vi "geve-generate_config_file.vi"(8 "error in (no error)":errorcluster) -> (0 "error out":errorcluster, 1 "serial cfg":T1={"timeout (ms)"=0, "VISA resource name"="", "baud rate"=0, "max expected byte count"=128}, 2 "info":string)   [LabVIEW 2018]
doc: "check if config file exists.\nif not create it ( also check if config folder exists) and populate default data.\nif exists, get the config."
uses:
  geve-serial_config_cluster.ctl
  <vilib>/Utility/config.llb/Write Key (String).vi
  <vilib>/Utility/config.llb/Write Key (I32).vi
  <vilib>/Utility/config.llb/Read Key (String).vi
  <vilib>/Utility/config.llb/Read Key (I32).vi
  <vilib>/Utility/config.llb/NI_LVConfig.lvlib
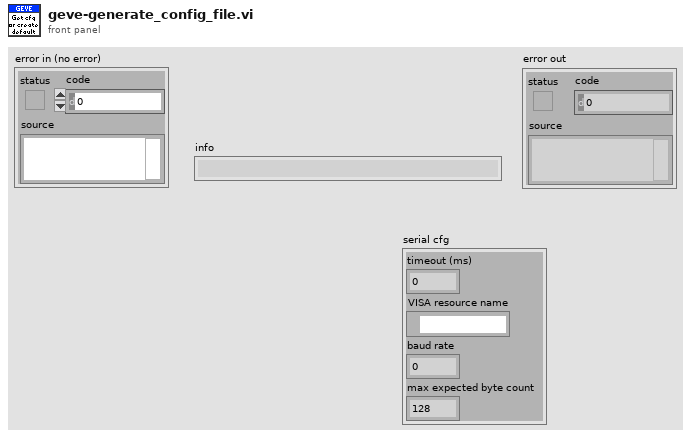
[diagram p1: front panel]
types:
  T1 = typedef "geve-serial_config_cluster.ctl" = cluster{"timeout (ms)":u32, "VISA resource name":refnum<visa-resource-name>, "baud rate":u32, "max expected byte count":u32}
  T2 = typedef "NI_LVConfig.lvlib/Config Data RefNum.ctl" = refnum<k1>
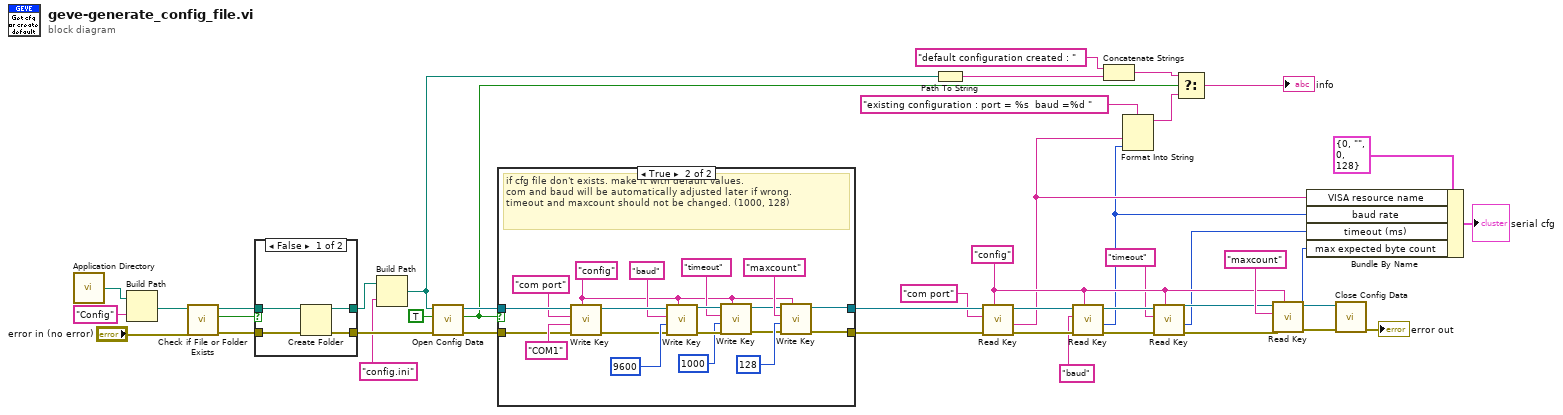
[diagram p0: block diagram]
diagram:
  w8 = "config" ("section")
  n1 = call <vilib>:"Application Directory.vi"() -> ("Application Directory"=w42:path)
  n2 = Build Path(base path=w42, name or relative path="Config") -> (appended path=w40:path)
  n3 = call <vilib>:"Check if File or Folder Exists.vi"("error in (no error)"="error in (no error)", "path"=w40) -> ("error out"=w35:errorcluster, "file or folder exists?"=w39:bool, "dup path"=w38:path)  [unwired: 7 in]
  n4 = case shown="False" w39 {
    tunnel: w38 -> [w47 w49]
    tunnel: [w46 w49] -> w26
    tunnel: [w44 w48] -> w36
    tunnel: w35 -> [w45 w48]
    frame False {
      n5 = Create Folder(path (use dialog)=w47, error in=w45) -> (created path=w46:path, error out=w44:errorcluster)  [unwired: 1 in, 1 out]
    }
    frame True {
    }
  }
  n6 = Build Path(base path=w26, name or relative path="config.ini") -> (appended path=w20:path)
  n7 = call <vilib>:"Open Config Data.vi"("error in (no error)"=w36, "create file if necessary (T)"=TRUE, "configuration file path"=w20) -> ("error out"=w33:errorcluster, "file created?"=w23:bool, "refnum"=w37:T2)  [unwired: 6 in]
  n8 = case shown="True" w23 {
    tunnel: w37 -> [w51 w70]
    tunnel: w33 -> [w50 w64]
    tunnel: [w51 w53] -> w31
    tunnel: [w50 w52] -> w30
    frame False {
    }
    frame True {
      w56 = "config" ("section")
      # "if cfg file don't exists. make it with default values.\ncom and baud will be automatically adjusted later if wrong.\ntimeout and maxcount should not be changed. (1000, 128)"
      n9 = call-poly <vilib>:"Write Key.vi"("section"=w56, "error in (no error)"=w64, "value"="COM1", "key"="com port", "refnum"=w70) -> ("error out"=w63:errorcluster, "refnum out"=w69:T2)  [unwired: 4 in, 1 out]
      n10 = call-poly <vilib>:"Write Key.vi"("section"=w56, "error in (no error)"=w63, "value"=9600, "key"="baud", "refnum"=w69) -> ("error out"=w61:errorcluster, "refnum out"=w62:T2)  [unwired: 4 in, 1 out]
      n11 = call-poly <vilib>:"Write Key.vi"("section"=w56, "error in (no error)"=w61, "value"=1000, "key"="timeout", "refnum"=w62) -> ("error out"=w55:errorcluster, "refnum out"=w54:T2)  [unwired: 4 in, 1 out]
      n12 = call-poly <vilib>:"Write Key.vi"("section"=w56, "error in (no error)"=w55, "value"=128, "key"="maxcount", "refnum"=w54) -> ("error out"=w52:errorcluster, "refnum out"=w53:T2)  [unwired: 4 in, 1 out]
    }
  }
  n13 = Path To String(path=w20) -> (string=w21:string)
  n14 = call-poly <vilib>:"Read Key.vi"("section"=w8, "error in (no error)"=w30, "key"="com port", "refnum"=w31) -> ("error out"=w29:errorcluster, "value"=w5:string, "refnum out"=w32:T2)  [unwired: 4 in, 1 out]
  n15 = call-poly <vilib>:"Read Key.vi"("section"=w8, "error in (no error)"=w29, "key"="baud", "refnum"=w32) -> ("error out"=w12:errorcluster, "value"=w4:i32, "refnum out"=w13:T2)  [unwired: 4 in, 1 out]
  n16 = Concatenate Strings("default configuration created : " ("section"), w21) -> (w19:string)
  n17 = Format Into String(format string="existing configuration : port = %s  baud =%d " ("section"), w5, w4) -> (resulting string=w17:string)  [unwired: 2 in, 1 out]
  n18 = call-poly <vilib>:"Read Key.vi"("section"=w8, "error in (no error)"=w12, "key"="timeout", "refnum"=w13) -> ("error out"=w11:errorcluster, "value"=w3:i32, "refnum out"=w14:T2)  [unwired: 4 in, 1 out]
  n19 = Select(t=w19, s=w23, f=w17) -> (s? t:f=→"info":string)
  n20 = call-poly <vilib>:"Read Key.vi"("section"=w8, "error in (no error)"=w11, "key"="maxcount", "refnum"=w14) -> ("error out"=w10:errorcluster, "value"=w2:i32, "refnum out"=w9:T2)  [unwired: 4 in, 1 out]
  n21 = Bundle By Name(cluster=T1 {"timeout (ms)"=0, "VISA resource name"="", "baud rate"=0, "max expected byte count"=128} ("Serial Port Configuration"), "VISA resource name"=w5, "baud rate"=w4, "timeout (ms)"=w3, "max expected byte count"=w2) -> (→"serial cfg":T1)
  n22 = call <vilib>:"Close Config Data.vi"("error in (no error)"=w10, "refnum"=w9) -> ("error out"=→"error out":errorcluster)  [unwired: 8 in, 1 out]
